vi "Format Variant Into String__ogtk.vi"(0 "Input String":string, 2 "format string":string, 7 "error in (no error)":errorcluster, 11 "Variant":variant) -> (4 "Output String":string, 8 "error out":errorcluster)   [LabVIEW 2011]
doc: "Overcomes a limitation of \"Format Into String\" by allowing variant data types to be used. This VI supports variant data for all LabVIEW data types supported by \"Format Into String\". The \"format string\" input may optionally be passed as an variant attribute named \"Format String\"."
panel:
  # "[OpenG VI Tags] ***Do Not Remove***"
  # "Format Variant Into String.vi\n\nOvercomes a limitation of \"Format Into String\" by allowing variant data types to be used.  This VI supports variant data for all LabVIEW data types supported by\n\"Format Into String\".  The \"format string\" input may optionally be passed as an variant attribute named \"Format String\"\n\nPlease visit http://www.OpenG.org to learn about the\nOpen Source LabVIEW software movement.\n\nNOTICE -- YOU MUST LEAVE THIS NOTICE IN PLACE.  PER THE TERMS OF THE LICENSE BELOW, YOU MAY SUBLICENSE THIS SOFTWARE \nIN ANY WAY THAT DOES NOT CONFLICT WITH THIS LICENSE.\n\n### BSD License (http://www.opensource.org/licenses/bsd-license.php) Begin ###\n \nCopyright (c) 2002-2004, Jim Kring <jim@jimkring.com>\nCopyright (c) 2004, Michael C. Ashe <michael.ashe@imaginatics.com>\n\nAll rights reserved.\n\nRedistribution and use in source and binary forms, with or without modification, are permitted provided that the following conditions are met:\n\n    * Redistributions of source code must retain the above copyright notice, this list of conditions and the following disclaimer.\n    * Redistributions in binary form must reproduce the above copyright notice, this list of conditions and the following disclaimer in the \n       documentation and/or other materials provided with the distribution.\n    * Neither the name of SciWare, James Kring, Inc., nor the names of its contributors may be used to endorse or promote products derived \n       from this software without specific prior written permission.\n\nTHIS SOFTWARE IS PROVIDED BY THE COPYRIGHT HOLDERS AND CONTRIBUTORS \"AS IS\" AND ANY EXPRESS OR IMPLIED WARRANTIES, \nINCLUDING, BUT NOT LIMITED TO, THE IMPLIED WARRANTIES OF MERCHANTABILITY AND FITNESS FOR A PARTICULAR PURPOSE ARE \nDISCLAIMED. IN NO EVENT SHALL THE COPYRIGHT OWNER OR CONTRIBUTORS BE LIABLE FOR ANY DIRECT, INDIRECT, INCIDENTAL,\n SPECIAL, EXEMPLARY, OR CONSEQUENTIAL DAMAGES (INCLUDING, BUT NOT LIMITED TO, PROCUREMENT OF SUBSTITUTE GOODS OR \nSERVICES; LOSS OF USE, DATA, OR PROFITS; OR BUSINESS INTERRUPTION) HOWEVER CAUSED AND ON ANY THEORY OF LIABILITY, \nWHETHER IN CONTRACT, STRICT LIABILITY, OR TORT (INCLUDING NEGLIGENCE OR OTHERWISE) ARISING IN ANY WAY OUT OF THE USE \nOF THIS SOFTWARE, EVEN IF ADVISED OF THE POSSIBILITY OF SUCH DAMAGE.\n\n### BSD License End ###"
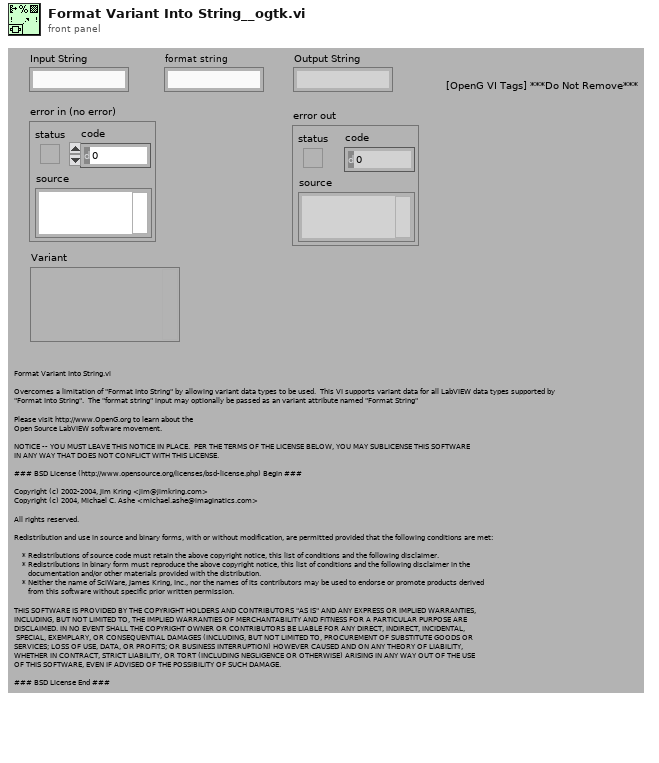
[diagram p1: front panel]
types:
  T1 = typedef "Type Descriptor Enumeration__ogtk.ctl" = enum8{"<Null>", "I8", "I16", "I32", "I64", "U8", "U16", "U32", "U64", "SGL", "DBL", "EXT", "CSG", "CDB", "CXT", "0x0F", "0x10", "0x11", "0x12", "0x13", "0x14", "Enum U8", "Enum U16", "Enum U32", "Enum U64", "SGL PQ", "DBL PQ", "EXT PQ", "CSG PQ", "CDB PQ", "CXT PQ", "0x1F", "0x20", "Boolean", "0x22", "0x23", "0x24", "0x25", "0x26", "0x27", "0x28", "0x29", "0x2A", "0x2B", "0x2C", "0x2D", "0x2E", "0x2F", "String", "0x31", "Path", "Pict", "0x34", "0x35", "0x36", "DAQ", "0x38", "0x39", "0x3A", "0x3B", "0x3C", "0x3D", "0x3E", "0x3F", "Array", "0x41", "0x42", "0x43", "0x44", "0x45", "0x46", "0x47", "0x48", "0x49", "0x4A", "0x4B", "0x4C", "0x4D", "0x4E", "0x4F", "Cluster", "0x51", "0x52", "Variant", "Waveform", "0x55", "0x56", "0x57", "0x58", "0x59", "0x5A", "0x5B", "0x5C", "0x5D", "0x5E", "0x5F", "0x60", "0x61", "0x62", "0x63", "0x64", "0x65", "0x66", "0x67", "0x68", "0x69", "0x6A", "0x6B", "0x6C", "0x6D", "0x6E", "0x6F", "Refnum"}
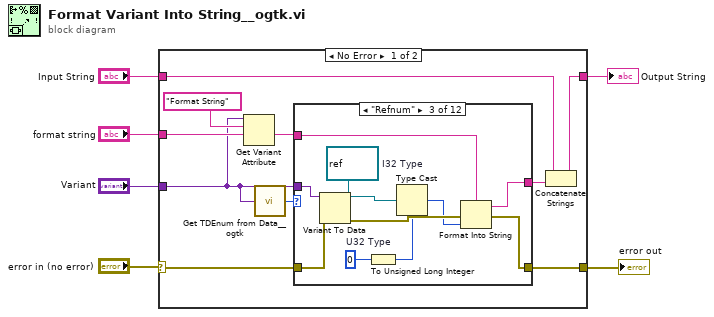
[diagram p0: block diagram]
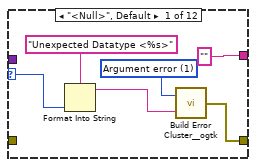
[diagram p2: hidden frame]
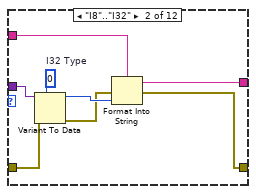
[diagram p3: hidden frame]
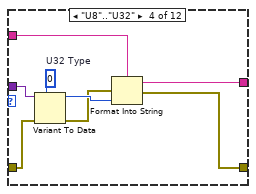
[diagram p4: hidden frame]
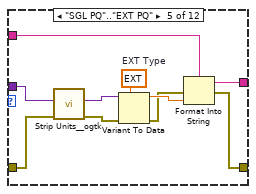
[diagram p5: hidden frame]
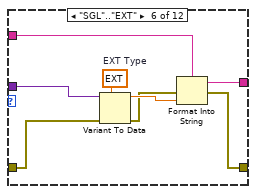
[diagram p6: hidden frame]
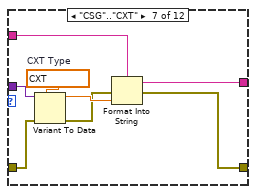
[diagram p7: hidden frame]
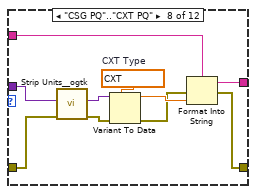
[diagram p8: hidden frame]
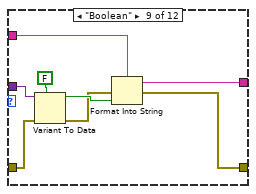
[diagram p9: hidden frame]
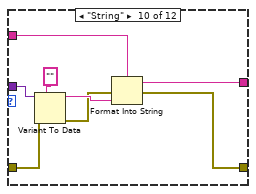
[diagram p10: hidden frame]
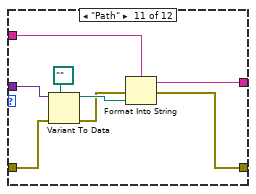
[diagram p11: hidden frame]
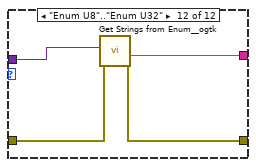
[diagram p12: hidden frame]
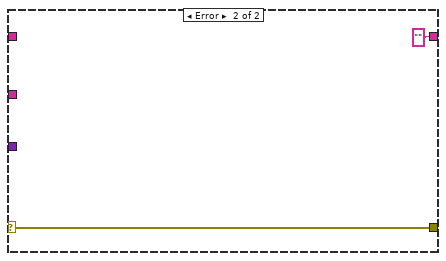
[diagram p13: hidden frame]
diagram:
  n1 = case shown="No Error" "error in (no error)" {
    selector: "error in (no error)" -> [w14 w115]
    tunnel: "Input String" -> [w11 _]
    tunnel: [w15 ""] -> w5
    tunnel: "format string" -> [w10 _]
    tunnel: "Variant" -> [w8 _]
    tunnel: [w13 w115] -> w1
    frame No Error {
      n2 = Get Variant Attribute(Variant=w8, name="Format String", default value (empty Variant)=w10) -> (value=w9:string)  [unwired: 1 in, 3 out]
      n3 = call "Get TDEnum from Data__ogtk.vi"("Data"=w8) -> ("Type Descriptor Enumeration"=w7:T1)  [unwired: 4 in]
      n4 = case shown="\"Refnum\"" w7 {
        selector: w7 -> [w18 _ _ _ _ _ _ _ _ _ _ _]
        tunnel: w8 -> [_ w29 w40 w48 w52 w61 w74 w78 w93 w101 w109 w113]
        tunnel: w9 -> [_ w27 w38 w46 w57 w65 w72 w83 w86 w99 w107 _]
        tunnel: ["" w26 w37 w45 w56 w64 w71 w82 w91 w98 w106 w111] -> w16
        tunnel: [w17 w23 w34 w42 w54 w62 w68 w80 w87 w95 w102 w110] -> w13
        tunnel: w14 -> [_ w25 w36 w44 w51 w60 w70 w77 w89 w94 w104 w112]
        frame "<Null>", Default {
          w21 = 1 items=["No error", "Argument error", "Memory is full", "Out of zone", "End of file", "File already open", "Generic file I/O error", "File not found", "File permission error", "Disk is full", "Duplicate path", "Too many files open", "System feature not enabled", "Resource file not found", "Cannot add resource", "Resource not found", "Image not found", "Image memory error", "Pen does not exist", "Config type invalid", "Config token not found", "Config parse error", "Config memory error", "Bad external code format", "Bad external code offset", "External code not present", "Null window", "Destroy window error", "Null menu", "Print aborted", "Bad print record", "Print driver error", "Windows error during printing", "Memory error during printing", "Print dialog error", "Generic print error", "Invalid device refnum", "Device not found", "Device parameter error", "Device unit error", "Cannot open device", "Device call aborted", "Generic error", "Cancelled by user", "Object ID too low", "Object ID too high", "Object not in heap", "Unknown heap", "Unknown object (invalid DefProc)", "Unknown object (DefProc not in table)", "Message out of range", "Invalid (null) method", "Unknown message", "Manager call not supported", "Bad address", "Network operation in progress", "Network operation timed out", "Connection is busy", "Network attribute not supported", "Network error", "Address in use", "System out of memory", "Connection aborted", "Connection refused", "Not connected", "Already connected", "Connection closed", "Initialization error (interapplication manager)", "Bad occurrence", "Wait on unbound occurrence handler", "Occurrence queue overflow", "Datalog type conflict", "Unused", "Unrecognized type (interapplication manager)", "Memory corrupt", "Failed to make temporary DLL", "Old CIN version", "Drag socket not found", "Failed to load drop-object", "Failed to register OLE object", "Failed to release OLE object", "Format specifier type mismatch", "Unknown format specifier", "Too few format specifiers", "Too many format specifiers", "Scan failed", "Newer CIN version", "Error converting to variant", "Runtime menu error", "Password tampered", "Variant attribute not found", "Incompatible variant data type", "Event data is not available", "Event Store is not present", "Occurrence is not found", "Event Queue is not created", "Event info is not available", "Refnum passed is NULL", "Error retrieving Class GUID", "Error retrieving CoClass GUID", "Error retrieving TypeLib GUID.", "Bad built application magic bytes.", "Specific driver is different from the specific driver associated with the Logical Name.", "There is no session opened to the class driver.", "Max Error", "MAX - Error with config objects", "MAX - Error loading configuration", "MAX - Group not supported"]
          n5 = Format Into String(format string="Unexpected Datatype <%s>" ("Format String"), w18) -> (resulting string=w19:string)  [unwired: 2 in, 1 out]
          n6 = call "Build Error Cluster__ogtk.vi"("String to Prepend to source (\"\")"=w19, "code"=w21) -> ("error out"=w17:errorcluster)
        }
        frame "I8".."I32" {
          w30 = 0  # I32 Type
          n7 = Variant To Data(error in=w25, type=w30, Variant=w29) -> (data=w28:i32, error out=w24:errorcluster)
          n8 = Format Into String(format string=w27, error in=w24, w28) -> (resulting string=w26:string, error out=w23:errorcluster)  [unwired: 1 in]
        }
        frame "Refnum" {
          w32 = u32 0  # U32 Type
          w41 = refnum<k0> refnum  # I32 Type
          n9 = Variant To Data(error in=w36, type=w41, Variant=w40) -> (data=w39:refnum<k0>, error out=w35:errorcluster)
          n10 = To Unsigned Long Integer(number=w32) -> (unsigned 32bit integer=w31:u32)
          n11 = Type Cast(type=w31, x=w39) -> (*(type *) &x=w33:u32)
          n12 = Format Into String(format string=w38, error in=w35, w33) -> (resulting string=w37:string, error out=w34:errorcluster)  [unwired: 1 in]
        }
        frame "U8".."U32" {
          w49 = u32 0  # U32 Type
          n13 = Variant To Data(error in=w44, type=w49, Variant=w48) -> (data=w47:u32, error out=w43:errorcluster)
          n14 = Format Into String(format string=w46, error in=w43, w47) -> (resulting string=w45:string, error out=w42:errorcluster)  [unwired: 1 in]
        }
        frame "SGL PQ".."EXT PQ" {
          w59 = ext 0.0  # EXT Type
          n15 = call "Strip Units__ogtk.vi"("error in (no error)"=w51, "Number or 1D array with units"=w52) -> ("error out"=w50:errorcluster, "Pure Number(s) (base units)"=w53:variant)  [unwired: 8 in]
          n16 = Variant To Data(error in=w50, type=w59, Variant=w53) -> (data=w58:ext, error out=w55:errorcluster)
          n17 = Format Into String(format string=w57, error in=w55, w58) -> (resulting string=w56:string, error out=w54:errorcluster)  [unwired: 1 in]
        }
        frame "SGL".."EXT" {
          w67 = ext 0.0  # EXT Type
          n18 = Variant To Data(error in=w60, type=w67, Variant=w61) -> (data=w66:ext, error out=w63:errorcluster)
          n19 = Format Into String(format string=w65, error in=w63, w66) -> (resulting string=w64:string, error out=w62:errorcluster)  [unwired: 1 in]
        }
        frame "CSG".."CXT" {
          w75 = cxt 0.0+0.0i  # CXT Type
          n20 = Variant To Data(error in=w70, type=w75, Variant=w74) -> (data=w73:cxt, error out=w69:errorcluster)
          n21 = Format Into String(format string=w72, error in=w69, w73) -> (resulting string=w71:string, error out=w68:errorcluster)  [unwired: 1 in]
        }
        frame "CSG PQ".."CXT PQ" {
          w85 = cxt 0.0+0.0i  # CXT Type
          n22 = call "Strip Units__ogtk.vi"("error in (no error)"=w77, "Number or 1D array with units"=w78) -> ("error out"=w76:errorcluster, "Pure Number(s) (base units)"=w79:variant)  [unwired: 8 in]
          n23 = Variant To Data(error in=w76, type=w85, Variant=w79) -> (data=w84:cxt, error out=w81:errorcluster)
          n24 = Format Into String(format string=w83, error in=w81, w84) -> (resulting string=w82:string, error out=w80:errorcluster)  [unwired: 1 in]
        }
        frame "Boolean" {
          n25 = Variant To Data(error in=w89, type=FALSE, Variant=w93) -> (data=w92:bool, error out=w88:errorcluster)
          n26 = Format Into String(format string=w86, error in=w88, w92) -> (resulting string=w91:string, error out=w87:errorcluster)  [unwired: 1 in]
        }
        frame "String" {
          n27 = Variant To Data(error in=w94, type="", Variant=w101) -> (data=w100:string, error out=w96:errorcluster)
          n28 = Format Into String(format string=w99, error in=w96, w100) -> (resulting string=w98:string, error out=w95:errorcluster)  [unwired: 1 in]
        }
        frame "Path" {
          n29 = Variant To Data(error in=w104, type=path "", Variant=w109) -> (data=w108:path, error out=w103:errorcluster)
          n30 = Format Into String(format string=w107, error in=w103, w108) -> (resulting string=w106:string, error out=w102:errorcluster)  [unwired: 1 in]
        }
        frame "Enum U8".."Enum U32" {
          n31 = call "Get Strings from Enum__ogtk.vi"("error in (no error)"=w112, "Enum"=w113) -> ("error out"=w110:errorcluster, "String Value"=w111:string)  [unwired: 6 in, 2 out]
        }
      }
      n32 = Concatenate Strings(w11, w16) -> (w15:string)
    }
    frame Error {
    }
  }
  "Output String" <- w5
  "error out" <- w1
